vi "Write Config.vi"(6 "Password":string="password", 7 "New File?":bool, 8 "error in (no error)":errorcluster, 10 "output cluster":T1={"LH"={"Go Up"={"Min Speed"=10.0, "Max Speed"=250.0, "Min Time"=0.5, "Max Time"=4.3, "Min Run Current"=0.0, "Max Run Current"=10.0, "Min Stall Current"=0.0, "Max Stall Current"=25.0, "Min Stall Force"=170.0, "Max Stall Force"=320.0, "Min Stroke"=254.4, "Max Stroke"=270.4}, "Go Down"={"Min Speed"=10.0, "Max Speed"=250.0, "Min Travel Time"=0.5, "Max Travel Time"=4.3, "Min Run Current"=0.0, "Max Run Current"=10.0}, "Shipping"={"Min Distance"=5.0, "Max Distance"=15.0, "Setpoint"=5.0}, "Anti-Pinch"={"Min Force"=0.0, "Max Force"=0.0}}, "RH"={"Go Up"={"Min Speed"=10.0, "Max Speed"=250.0, "Min Time"=0.5, "Max Time"=4.3, "Min Run Current"=0.0, "Max Run Current"=10.0, "Min Stall Current"=0.0, "Max Stall Current"=25.0, "Min Stall Force"=170.0, "Max Stall Force"=320.0, "Min Stroke"=254.4, "Max Stroke"=270.4}, "Go Down"={"Min Speed"=10.0, "Max Speed"=250.0, "Min Travel Time"=0.5, "Max Travel Time"=4.3, "Min Run Current"=0.0, "Max Run Current"=10.0}, "Shipping"={"Min Distance"=5.0, "Max Distance"=15.0, "Setpoint"=5.0}, "Anti-Pinch"={"Min Force"=0.0, "Max Force"=0.0}}, "W 601 FR RH Std"={"Go Up"={"Min Speed"=0.0, "Max Speed"=0.0, "Min Time"=2.0, "Max Time"=5.0, "Min Run Current"=0.0, "Max Run Current"=9.0, "Min Stall Current"=0.0, "Max Stall Current"=25.0, "Min Stall Force"=200.0, "Max Stall Force"=350.0, "Min Stroke"=0.0, "Max Stroke"=465.9}, "Go Down"={"Min Speed"=0.0, "Max Speed"=0.0, "Min Travel Time"=2.0, "Max Travel Time"=5.0, "Min Run Current"=0.0, "Max Run Current"=9.0}, "Shipping"={"Min Distance"=80.6, "Max Distance"=100.6, "Setpoint"=0.0}, "Anti-Pinch"={"Min Force"=0.0, "Max Force"=0.0}}, "W 601 FR LH Std"={"Go Up"={"Min Speed"=0.0, "Max Speed"=0.0, "Min Time"=2.0, "Max Time"=5.0, "Min Run Current"=0.0, "Max Run Current"=9.0, "Min Stall Current"=0.0, "Max Stall Current"=25.0, "Min Stall Force"=200.0, "Max Stall Force"=350.0, "Min Stroke"=0.0, "Max Stroke"=465.9}, "Go Down"={"Min Speed"=0.0, "Max Speed"=0.0, "Min Travel Time"=2.0, "Max Travel Time"=5.0, "Min Run Current"=0.0, "Max Run Current"=9.0}, "Shipping"={"Min Distance"=80.6, "Max Distance"=100.6, "Setpoint"=0.0}, "Anti-Pinch"={"Min Force"=0.0, "Max Force"=0.0}}, "W 601 RR RH Std"={"Go Up"={"Min Speed"=0.0, "Max Speed"=0.0, "Min Time"=2.0, "Max Time"=5.0, "Min Run Current"=0.0, "Max Run Current"=9.0, "Min Stall Current"=0.0, "Max Stall Current"=25.0, "Min Stall Force"=150.0, "Max Stall Force"=300.0, "Min Stroke"=0.0, "Max Stroke"=450.7}, "Go Down"={"Min Speed"=0.0, "Max Speed"=0.0, "Min Travel Time"=2.0, "Max Travel Time"=5.0, "Min Run Current"=0.0, "Max Run Current"=9.0}, "Shipping"={"Min Distance"=83.0, "Max Distance"=103.0, "Setpoint"=0.0}, "Anti-Pinch"={"Min Force"=0.0, "Max Force"=0.0}}, "W 601 RR LH Std"={"Go Up"={"Min Speed"=0.0, "Max Speed"=0.0, "Min Time"=2.0, "Max Time"=5.0, "Min Run Current"=0.0, "Max Run Current"=9.0, "Min Stall Current"=0.0, "Max Stall Current"=25.0, "Min Stall Force"=150.0, "Max Stall Force"=300.0, "Min Stroke"=0.0, "Max Stroke"=450.7}, "Go Down"={"Min Speed"=0.0, "Max Speed"=0.0, "Min Travel Time"=2.0, "Max Travel Time"=5.0, "Min Run Current"=0.0, "Max Run Current"=9.0}, "Shipping"={"Min Distance"=83.0, "Max Distance"=103.0, "Setpoint"=0.0}, "Anti-Pinch"={"Min Force"=0.0, "Max Force"=0.0}}, "W 601 FR RH AP"={"Go Up"={"Min Speed"=0.0, "Max Speed"=0.0, "Min Time"=2.0, "Max Time"=5.0, "Min Run Current"=0.0, "Max Run Current"=9.0, "Min Stall Current"=0.0, "Max Stall Current"=25.0, "Min Stall Force"=200.0, "Max Stall Force"=350.0, "Min Stroke"=0.0, "Max Stroke"=465.9}, "Go Down"={"Min Speed"=0.0, "Max Speed"=0.0, "Min Travel Time"=2.0, "Max Travel Time"=5.0, "Min Run Current"=0.0, "Max Run Current"=9.0}, "Shipping"={"Min Distance"=80.6, "Max Distance"=100.6, "Setpoint"=0.0}, "Anti-Pinch"={"Min Force"=0.0, "Max Force"=100.0}}, "W 601 FR LH AP"={"Go Up"={"Min Speed"=0.0, "Max Speed"=0.0, "Min Time"=2.0, "Max Time"=5.0, "Min Run Current"=0.0, "Max Run Current"=9.0, "Min Stall Current"=0.0, "Max Stall Current"=25.0, "Min Stall Force"=200.0, "Max Stall Force"=350.0, "Min Stroke"=0.0, "Max Stroke"=465.9}, "Go Down"={"Min Speed"=0.0, "Max Speed"=0.0, "Min Travel Time"=2.0, "Max Travel Time"=5.0, "Min Run Current"=0.0, "Max Run Current"=9.0}, "Shipping"={"Min Distance"=80.6, "Max Distance"=100.6, "Setpoint"=0.0}, "Anti-Pinch"={"Min Force"=0.0, "Max Force"=100.0}}, "W 601 RR RH AP"={"Go Up"={"Min Speed"=0.0, "Max Speed"=0.0, "Min Time"=2.0, "Max Time"=5.0, "Min Run Current"=0.0, "Max Run Current"=9.0, "Min Stall Current"=0.0, "Max Stall Current"=25.0, "Min Stall Force"=150.0, "Max Stall Force"=300.0, "Min Stroke"=0.0, "Max Stroke"=450.7}, "Go Down"={"Min Speed"=0.0, "Max Speed"=0.0, "Min Travel Time"=2.0, "Max Travel Time"=5.0, "Min Run Current"=0.0, "Max Run Current"=9.0}, "Shipping"={"Min Distance"=83.0, "Max Distance"=103.0, "Setpoint"=0.0}, "Anti-Pinch"={"Min Force"=0.0, "Max Force"=100.0}}, "W 601 RR LH AP"={"Go Up"={"Min Speed"=0.0, "Max Speed"=0.0, "Min Time"=2.0, "Max Time"=5.0, "Min Run Current"=0.0, "Max Run Current"=9.0, "Min Stall Current"=0.0, "Max Stall Current"=25.0, "Min Stall Force"=150.0, "Max Stall Force"=300.0, "Min Stroke"=0.0, "Max Stroke"=450.7}, "Go Down"={"Min Speed"=0.0, "Max Speed"=0.0, "Min Travel Time"=2.0, "Max Travel Time"=5.0, "Min Run Current"=0.0, "Max Run Current"=9.0}, "Shipping"={"Min Distance"=83.0, "Max Distance"=103.0, "Setpoint"=0.0}, "Anti-Pinch"={"Min Force"=0.0, "Max Force"=100.0}}}, 11 "file path":path=path "C:/Project/20-020_W601/trunk/config.ini") -> (0 "error out":errorcluster, 3 "file path out":path)   [LabVIEW 2017]
doc: "v1.1:\n- Added SenseON Delay\n\nv1.0:\n- Added 2WR bool"
uses:
  controls/All Specs.ctl
  controls/Specifications.ctl
  <vilib>/Utility/config.llb/Write Key (Double).vi
  <vilib>/Utility/config.llb/Write Key (String).vi
  <vilib>/Utility/config.llb/NI_LVConfig.lvlib
panel:
  in  "code":i32
  out "file created?":bool
  in  "Shipping":dbl=100.1 format="%#_13g"
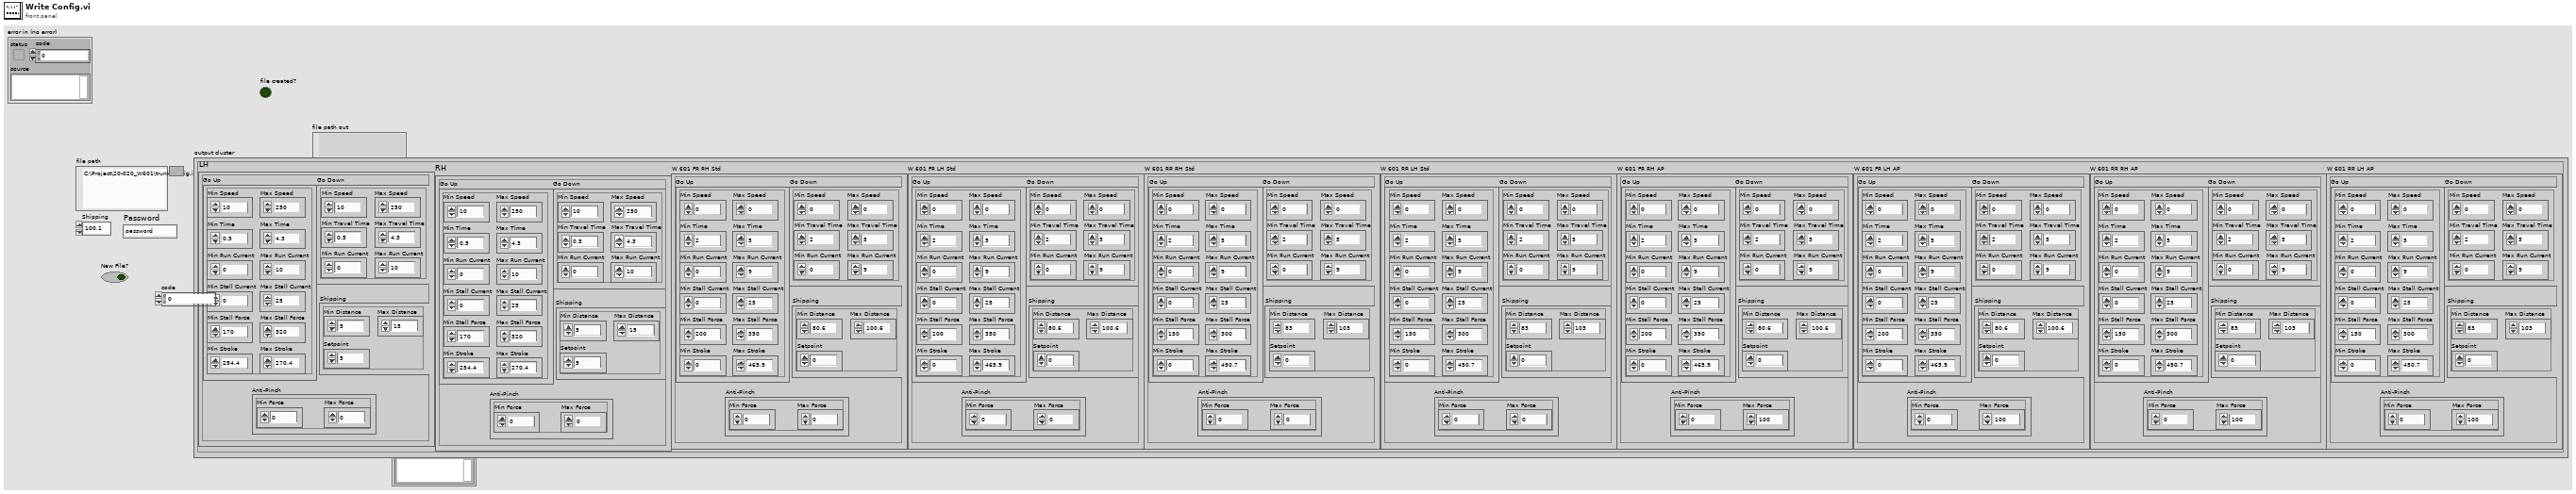
[diagram p1: front panel]
types:
  T1 = typedef "All Specs.ctl" = cluster{"LH":T2, "RH":T2, "W 601 FR RH Std":T2, "W 601 FR LH Std":T2, "W 601 RR RH Std":T2, "W 601 RR LH Std":T2, "W 601 FR RH AP":T2, "W 601 FR LH AP":T2, "W 601 RR RH AP":T2, "W 601 RR LH AP":T2}
  T2 = typedef "Specifications.ctl" = cluster{"Go Up":cluster{"Min Speed":dbl, "Max Speed":dbl, "Min Time":dbl, "Max Time":dbl, "Min Run Current":dbl, "Max Run Current":dbl, "Min Stall Current":dbl, "Max Stall Current":dbl, "Min Stall Force":dbl, "Max Stall Force":dbl, "Min Stroke":dbl, "Max Stroke":dbl}, "Go Down":cluster{"Min Speed":dbl, "Max Speed":dbl, "Min Travel Time":dbl, "Max Travel Time":dbl, "Min Run Current":dbl, "Max Run Current":dbl}, "Shipping":cluster{"Min Distance":dbl, "Max Distance":dbl, "Setpoint":dbl}, "Anti-Pinch":cluster{"Min Force":dbl, "Max Force":dbl}}
  T3 = typedef "NI_LVConfig.lvlib/Config Data RefNum.ctl" = refnum<k1>
  T4 = cluster{"Min Speed":dbl, "Max Speed":dbl, "Min Time":dbl, "Max Time":dbl, "Min Run Current":dbl, "Max Run Current":dbl, "Min Stall Current":dbl, "Max Stall Current":dbl, "Min Stall Force":dbl, "Max Stall Force":dbl, "Min Stroke":dbl, "Max Stroke":dbl}
  T5 = cluster{"Min Speed":dbl, "Max Speed":dbl, "Min Travel Time":dbl, "Max Travel Time":dbl, "Min Run Current":dbl, "Max Run Current":dbl}
  T6 = cluster{"Min Distance":dbl, "Max Distance":dbl, "Setpoint":dbl}
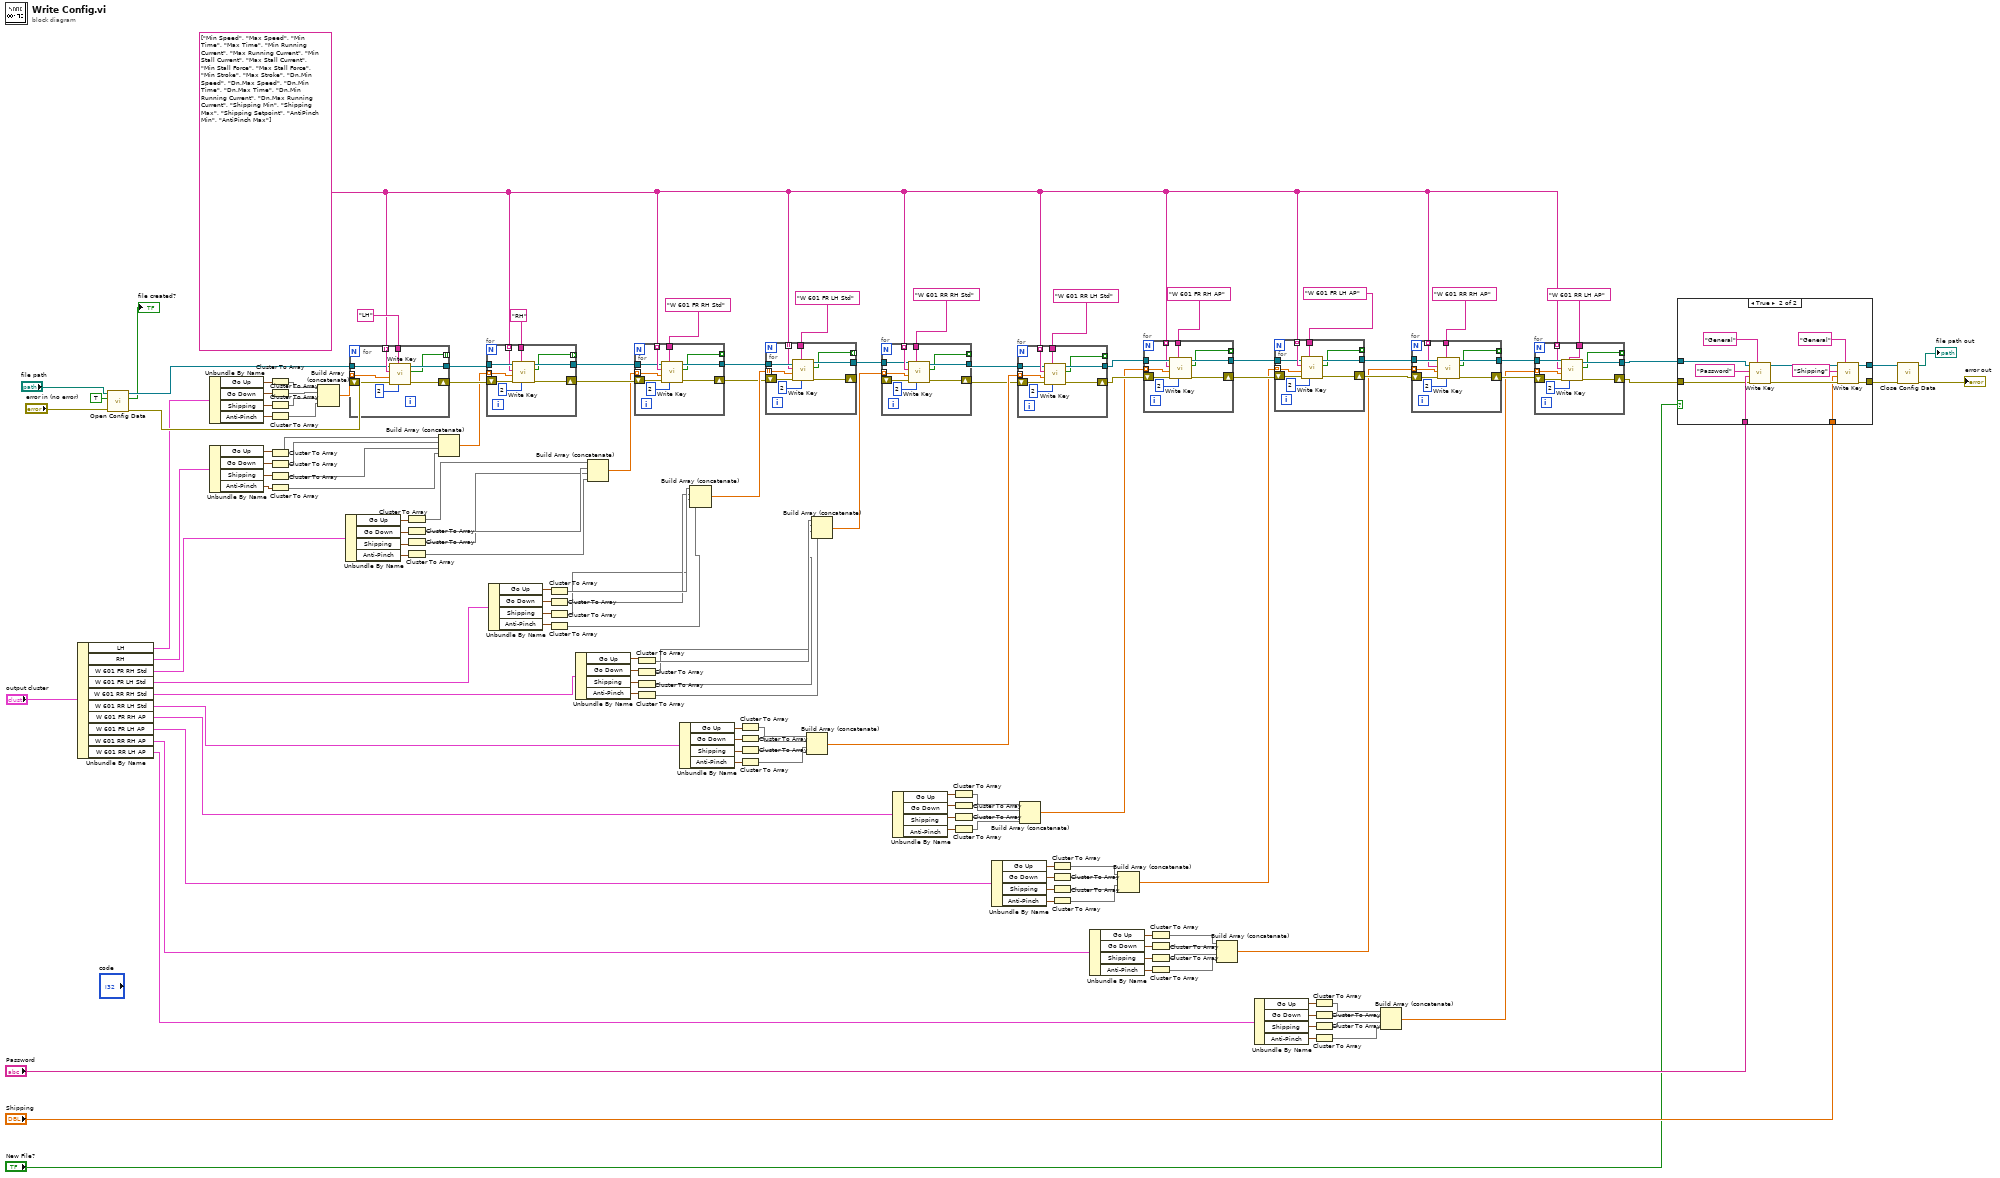
[diagram p0: block diagram]
diagram:
  w9 = string[] ["Min Speed", "Max Speed", "Min Time", "Max Time", "Min Running Current", "Max Running Current", "Min Stall Current", "Max Stall Current", "Min Stall Force", "Max Stall Force", "Min Stroke", "Max Stroke", "Dn.Min Speed", "Dn.Max Speed", "Dn.Min Time", "Dn.Max Time", "Dn.Min Running Current", "Dn.Max Running Current", "Shipping Min", "Shipping Max", "Shipping Setpoint", "AntiPinch Min", "AntiPinch Max"]
  n1 = Unbundle By Name("output cluster") -> ("LH"=w110:T2, "RH"=w109:T2, "W 601 FR RH Std"=w108:T2, "W 601 FR LH Std"=w107:T2, "W 601 RR RH Std"=w106:T2, "W 601 RR LH Std"=w105:T2, "W 601 FR RH AP"=w104:T2, "W 601 FR LH AP"=w103:T2, "W 601 RR RH AP"=w102:T2, "W 601 RR LH AP"=w101:T2)
  n2 = call <vilib>:"Open Config Data.vi"("error in (no error)"="error in (no error)", "create file if necessary (T)"=TRUE, "configuration file path"="file path") -> ("error out"=w122:errorcluster, "file created?"=→"file created?":bool, "refnum"=w117:T3)  [unwired: 6 in]
  n3 = Unbundle By Name(w110) -> ("Go Up"=w136:T4, "Go Down"=w135:T5, "Shipping"=w134:T6, "Anti-Pinch"=w112:cluster{"Min Force":dbl, "Max Force":dbl})
  n4 = Unbundle By Name(w109) -> ("Go Up"=w133:T4, "Go Down"=w132:T5, "Shipping"=w131:T6, "Anti-Pinch"=w114:cluster{"Min Force":dbl, "Max Force":dbl})
  n5 = Cluster To Array(cluster=w136) -> (array=w130:dbl[])
  n6 = Cluster To Array(cluster=w135) -> (array=w129:dbl[])
  n7 = Cluster To Array(cluster=w134) -> (array=w128:dbl[])
  n8 = Cluster To Array(cluster=w112) -> (array=w111:dbl[])
  n9 = Cluster To Array(cluster=w133) -> (array=w126:dbl[])
  n10 = Cluster To Array(cluster=w132) -> (array=w125:dbl[])
  n11 = Cluster To Array(cluster=w131) -> (array=w124:dbl[])
  n12 = Cluster To Array(cluster=w114) -> (array=w113:dbl[])
  n13 = Build Array (concatenate)(w130, w129, w128, w111) -> (w127:dbl[])
  n14 = Unbundle By Name(w108) -> ("Go Up"=w100:T4, "Go Down"=w99:T5, "Shipping"=w98:T6, "Anti-Pinch"=w97:cluster{"Min Force":dbl, "Max Force":dbl})
  n15 = for {
    tunnel: "LH" ("section") -> [w152]
    tunnel: [w151] -> w139
    shift-right: [w150] -> w140
    shift-left: w122 -> [w153]
    tunnel: [w149] -> _ mode=indexing
    tunnel: w9 -> [w147] mode=indexing
    tunnel: w127 -> [w146] mode=indexing
    tunnel: w117 -> [w145]
    n16 = call-poly <vilib>:"Write Key.vi"("precision (6)"=i16 2, "section"=w152, "error in (no error)"=w153, "value"=w146, "key"=w147, "refnum"=w145) -> ("error out"=w150:errorcluster, "found?"=w149:bool, "refnum out"=w151:T3)  [unwired: 3 in]
  }
  n17 = Cluster To Array(cluster=w100) -> (array=w68:dbl[])
  n18 = Cluster To Array(cluster=w99) -> (array=w67:dbl[])
  n19 = Cluster To Array(cluster=w98) -> (array=w66:dbl[])
  n20 = Cluster To Array(cluster=w97) -> (array=w65:dbl[])
  n21 = Build Array (concatenate)(w126, w125, w124, w113) -> (w123:dbl[])
  n22 = for {
    tunnel: w139 -> [w161]
    tunnel: "RH" ("section") -> [w160]
    shift-right: [w159] -> w35
    shift-left: w140 -> [w162]
    tunnel: [w158] -> w36
    tunnel: [w157] -> _ mode=indexing
    tunnel: w9 -> [w155] mode=indexing
    tunnel: w123 -> [w154] mode=indexing
    n23 = call-poly <vilib>:"Write Key.vi"("precision (6)"=i16 2, "section"=w160, "error in (no error)"=w162, "value"=w154, "key"=w155, "refnum"=w161) -> ("error out"=w159:errorcluster, "found?"=w157:bool, "refnum out"=w158:T3)  [unwired: 3 in]
  }
  n24 = Unbundle By Name(w107) -> ("Go Up"=w69:T4, "Go Down"=w70:T5, "Shipping"=w71:T6, "Anti-Pinch"=w72:cluster{"Min Force":dbl, "Max Force":dbl})
  n25 = Cluster To Array(cluster=w69) -> (array=w64:dbl[])
  n26 = Cluster To Array(cluster=w70) -> (array=w63:dbl[])
  n27 = Cluster To Array(cluster=w71) -> (array=w62:dbl[])
  n28 = Cluster To Array(cluster=w72) -> (array=w61:dbl[])
  n29 = Unbundle By Name(w106) -> ("Go Up"=w96:T4, "Go Down"=w95:T5, "Shipping"=w94:T6, "Anti-Pinch"=w93:cluster{"Min Force":dbl, "Max Force":dbl})
  n30 = Build Array (concatenate)(w68, w67, w66, w65) -> (w34:dbl[])
  n31 = for {
    shift-right: [w170] -> w31
    shift-left: w35 -> [w171]
    tunnel: [w169] -> w30
    tunnel: [w168] -> _ mode=indexing
    tunnel: w9 -> [w166] mode=indexing
    tunnel: w36 -> [w165]
    tunnel: w34 -> [w164] mode=indexing
    tunnel: "W 601 FR RH Std" -> [w163]
    n32 = call-poly <vilib>:"Write Key.vi"("precision (6)"=i16 2, "section"=w163, "error in (no error)"=w171, "value"=w164, "key"=w166, "refnum"=w165) -> ("error out"=w170:errorcluster, "found?"=w168:bool, "refnum out"=w169:T3)  [unwired: 3 in]
  }
  n33 = Cluster To Array(cluster=w96) -> (array=w60:dbl[])
  n34 = Cluster To Array(cluster=w95) -> (array=w59:dbl[])
  n35 = Cluster To Array(cluster=w94) -> (array=w58:dbl[])
  n36 = Cluster To Array(cluster=w93) -> (array=w57:dbl[])
  n37 = Unbundle By Name(w105) -> ("Go Up"=w92:T4, "Go Down"=w91:T5, "Shipping"=w90:T6, "Anti-Pinch"=w89:cluster{"Min Force":dbl, "Max Force":dbl})
  n38 = Build Array (concatenate)(w64, w63, w62, w61) -> (w32:dbl[])
  n39 = Cluster To Array(cluster=w92) -> (array=w56:dbl[])
  n40 = Cluster To Array(cluster=w91) -> (array=w55:dbl[])
  n41 = Cluster To Array(cluster=w90) -> (array=w54:dbl[])
  n42 = Cluster To Array(cluster=w89) -> (array=w53:dbl[])
  n43 = for {
    shift-right: [w179] -> _
    shift-left: w31 -> [w180]
    tunnel: [w178] -> w3
    tunnel: [w177] -> _ mode=indexing
    tunnel: w32 -> [w175] mode=indexing
    tunnel: w30 -> [w174]
    tunnel: w9 -> [w173] mode=indexing
    tunnel: "W 601 FR LH Std" -> [w172]
    n44 = call-poly <vilib>:"Write Key.vi"("precision (6)"=i16 2, "section"=w172, "error in (no error)"=w180, "value"=w175, "key"=w173, "refnum"=w174) -> ("error out"=w179:errorcluster, "found?"=w177:bool, "refnum out"=w178:T3)  [unwired: 3 in]
  }
  n45 = Build Array (concatenate)(w56, w55, w54, w53) -> (w25:dbl[])
  n46 = Build Array (concatenate)(w60, w59, w58, w57) -> (w27:dbl[])
  n47 = for {
    shift-right: [w188] -> w23
    shift-left: _ -> [w189]
    tunnel: [w187] -> w24
    tunnel: [w186] -> _ mode=indexing
    tunnel: w9 -> [w184] mode=indexing
    tunnel: "W 601 RR RH Std" -> [w183]
    tunnel: w27 -> [w182] mode=indexing
    tunnel: w3 -> [w181]
    n48 = call-poly <vilib>:"Write Key.vi"("precision (6)"=i16 2, "section"=w183, "error in (no error)"=w189, "value"=w182, "key"=w184, "refnum"=w181) -> ("error out"=w188:errorcluster, "found?"=w186:bool, "refnum out"=w187:T3)  [unwired: 3 in]
  }
  n49 = Unbundle By Name(w104) -> ("Go Up"=w88:T4, "Go Down"=w87:T5, "Shipping"=w86:T6, "Anti-Pinch"=w85:cluster{"Min Force":dbl, "Max Force":dbl})
  n50 = Cluster To Array(cluster=w88) -> (array=w52:dbl[])
  n51 = Cluster To Array(cluster=w87) -> (array=w51:dbl[])
  n52 = Cluster To Array(cluster=w86) -> (array=w50:dbl[])
  n53 = Cluster To Array(cluster=w85) -> (array=w49:dbl[])
  n54 = Unbundle By Name(w103) -> ("Go Up"=w84:T4, "Go Down"=w83:T5, "Shipping"=w82:T6, "Anti-Pinch"=w81:cluster{"Min Force":dbl, "Max Force":dbl})
  n55 = for {
    shift-right: [w197] -> w22
    shift-left: w23 -> [w198]
    tunnel: [w196] -> w21
    tunnel: [w195] -> _ mode=indexing
    tunnel: w9 -> [w193] mode=indexing
    tunnel: "W 601 RR LH Std" -> [w192]
    tunnel: w25 -> [w191] mode=indexing
    tunnel: w24 -> [w190]
    n56 = call-poly <vilib>:"Write Key.vi"("precision (6)"=i16 2, "section"=w192, "error in (no error)"=w198, "value"=w191, "key"=w193, "refnum"=w190) -> ("error out"=w197:errorcluster, "found?"=w195:bool, "refnum out"=w196:T3)  [unwired: 3 in]
  }
  n57 = Build Array (concatenate)(w52, w51, w50, w49) -> (w19:dbl[])
  n58 = Cluster To Array(cluster=w84) -> (array=w48:dbl[])
  n59 = Cluster To Array(cluster=w83) -> (array=w47:dbl[])
  n60 = Cluster To Array(cluster=w82) -> (array=w46:dbl[])
  n61 = Cluster To Array(cluster=w81) -> (array=w45:dbl[])
  n62 = Unbundle By Name(w102) -> ("Go Up"=w80:T4, "Go Down"=w79:T5, "Shipping"=w78:T6, "Anti-Pinch"=w77:cluster{"Min Force":dbl, "Max Force":dbl})
  n63 = Build Array (concatenate)(w48, w47, w46, w45) -> (w16:dbl[])
  n64 = for {
    shift-right: [w206] -> w17
    shift-left: w22 -> [w207]
    tunnel: [w205] -> w18
    tunnel: [w204] -> _ mode=indexing
    tunnel: w21 -> [w202]
    tunnel: w9 -> [w201] mode=indexing
    tunnel: "W 601 FR RH AP" -> [w200]
    tunnel: w19 -> [w199] mode=indexing
    n65 = call-poly <vilib>:"Write Key.vi"("precision (6)"=i16 2, "section"=w200, "error in (no error)"=w207, "value"=w199, "key"=w201, "refnum"=w202) -> ("error out"=w206:errorcluster, "found?"=w204:bool, "refnum out"=w205:T3)  [unwired: 3 in]
  }
  n66 = Cluster To Array(cluster=w80) -> (array=w44:dbl[])
  n67 = Cluster To Array(cluster=w79) -> (array=w43:dbl[])
  n68 = Cluster To Array(cluster=w78) -> (array=w42:dbl[])
  n69 = Cluster To Array(cluster=w77) -> (array=w41:dbl[])
  n70 = Build Array (concatenate)(w44, w43, w42, w41) -> (w12:dbl[])
  n71 = Unbundle By Name(w101) -> ("Go Up"=w76:T4, "Go Down"=w75:T5, "Shipping"=w74:T6, "Anti-Pinch"=w73:cluster{"Min Force":dbl, "Max Force":dbl})
  n72 = for {
    shift-right: [w215] -> w13
    shift-left: w17 -> [w216]
    tunnel: [w214] -> w14
    tunnel: [w213] -> _ mode=indexing
    tunnel: w9 -> [w211] mode=indexing
    tunnel: w18 -> [w210]
    tunnel: w16 -> [w209] mode=indexing
    tunnel: "W 601 FR LH AP" -> [w208]
    n73 = call-poly <vilib>:"Write Key.vi"("precision (6)"=i16 2, "section"=w208, "error in (no error)"=w216, "value"=w209, "key"=w211, "refnum"=w210) -> ("error out"=w215:errorcluster, "found?"=w213:bool, "refnum out"=w214:T3)  [unwired: 3 in]
  }
  n74 = Cluster To Array(cluster=w76) -> (array=w40:dbl[])
  n75 = Cluster To Array(cluster=w75) -> (array=w39:dbl[])
  n76 = Cluster To Array(cluster=w74) -> (array=w38:dbl[])
  n77 = Cluster To Array(cluster=w73) -> (array=w37:dbl[])
  n78 = Build Array (concatenate)(w40, w39, w38, w37) -> (w8:dbl[])
  n79 = for {
    shift-right: [w224] -> w11
    shift-left: w13 -> [w225]
    tunnel: [w223] -> w10
    tunnel: [w222] -> _ mode=indexing
    tunnel: w14 -> [w220]
    tunnel: w9 -> [w219] mode=indexing
    tunnel: w12 -> [w218] mode=indexing
    tunnel: "W 601 RR RH AP" -> [w217]
    n80 = call-poly <vilib>:"Write Key.vi"("precision (6)"=i16 2, "section"=w217, "error in (no error)"=w225, "value"=w218, "key"=w219, "refnum"=w220) -> ("error out"=w224:errorcluster, "found?"=w222:bool, "refnum out"=w223:T3)  [unwired: 3 in]
  }
  n81 = for {
    shift-right: [w233] -> w6
    shift-left: w11 -> [w234]
    tunnel: [w232] -> w7
    tunnel: [w231] -> _ mode=indexing
    tunnel: w10 -> [w230]
    tunnel: w9 -> [w229] mode=indexing
    tunnel: w8 -> [w228] mode=indexing
    tunnel: "W 601 RR LH AP" -> [w227]
    n82 = call-poly <vilib>:"Write Key.vi"("precision (6)"=i16 2, "section"=w227, "error in (no error)"=w234, "value"=w228, "key"=w229, "refnum"=w230) -> ("error out"=w233:errorcluster, "found?"=w231:bool, "refnum out"=w232:T3)  [unwired: 3 in]
  }
  n83 = case shown="True" "New File?" {
    tunnel: [w236 w242] -> w121
    tunnel: [w235 w241] -> w120
    tunnel: "Password" -> [_ w240]
    tunnel: "Shipping" -> [_ w239]
    tunnel: w7 -> [w236 w238]
    tunnel: w6 -> [w235 w237]
    frame False {
    }
    frame True {
      n84 = call-poly <vilib>:"Write Key.vi"("section"="General", "error in (no error)"=w237, "value"=w240, "key"="Password", "refnum"=w238) -> ("error out"=w243:errorcluster, "refnum out"=w244:T3)  [unwired: 4 in, 1 out]
      n85 = call-poly <vilib>:"Write Key.vi"("section"="General", "error in (no error)"=w243, "value"=w239, "key"="Shipping", "refnum"=w244) -> ("error out"=w241:errorcluster, "refnum out"=w242:T3)  [unwired: 4 in, 1 out]
    }
  }
  n86 = call <vilib>:"Close Config Data.vi"("error in (no error)"=w120, "refnum"=w121) -> ("error out"=→"error out":errorcluster, "file path"=→"file path out":path)  [unwired: 8 in]
